vi "Store Websocket Refs.vi"(10 "WebSocket in":refnum<class "WebSocket.lvclass">, 11 "menu":T1(ring)=enum."remove client") -> (2 "Clients":refnum<class "WebSocket.lvclass">[](array[class]))   [LabVIEW 2019]
uses:
  <vilib>/mediamongrels ltd/websockets/websockets/websocket/WebSocket.lvclass
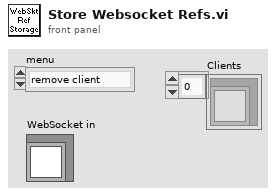
[diagram p1: front panel]
types:
  T1 = enum16{"add client", "remove client", "get clients", "clear"}
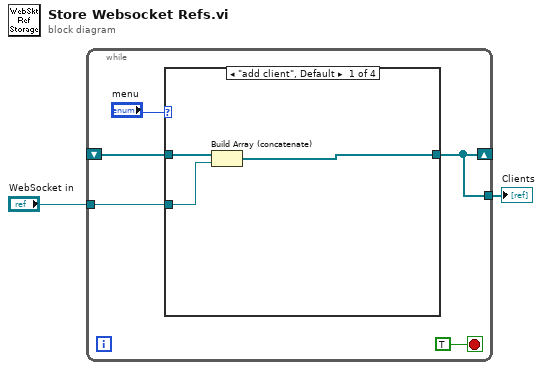
[diagram p0: block diagram]
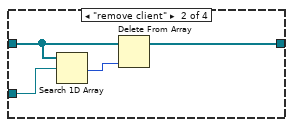
[diagram p2: hidden frame]
diagram:
  n1 = while {
    shift-right: [w3] -> _
    shift-left: _ -> [w5]
    tunnel: "WebSocket in" -> [w4]
    tunnel: [w3] -> w1
    stop <- TRUE stop-if-true
    n2 = case shown="\"add client\", Default" "menu" {
      tunnel: w5 -> [w9 w13 w15 _]
      tunnel: w4 -> [w10 w12 _ _]
      tunnel: [w8 w14 w15 _] -> w3
      frame "add client", Default {
        n3 = Build Array (concatenate)(w9, w10) -> (w8:refnum<class "WebSocket.lvclass">[])
      }
      frame "remove client" {
        n4 = Search 1D Array(1D array=w13, element=w12) -> (index of element=w11:i32)  [unwired: 1 in]
        n5 = Delete From Array(array=w13, index=w11) -> (array with subset deleted=w14:refnum<class "WebSocket.lvclass">[])  [unwired: 1 in, 1 out]
      }
      frame "get clients" {
      }
      frame "clear" {
      }
    }
  }
  "Clients" <- w1
